vi "DENSITY_txt.vi"(1 "uL/stroke":dbl=5.896, 5 "GUID":string, 7 "derate":dbl=1.0, 9 "Prime":bool=TRUE) -> (3 "density (g/mL)":dbl, 4 "mean":dbl format="%0.4f", 6 "mean 2":dbl format="%0.4f", 8 "standard deviation":dbl format="%0.4f", 10 "standard deviation 2":dbl format="%0.4f", 14 "xxx":bool[](array[boolean]), 15 "Err?":string)   [LabVIEW 2019]
uses:
  <vilib>/Analysis/NI_AALBase.lvlib
panel:
  out "sample (g)":dbl[](array[numeric])
  out "variance 2":dbl format="%0.4f"
  out "InvalidCommandErr? 2":bool
  out "tare (g)":dbl[](array[numeric])
  out "variance":dbl format="%0.4f"
  out "InvalidCommandErr?":bool
  out "log_string":string
  out "SampleVolume (mL)":dbl
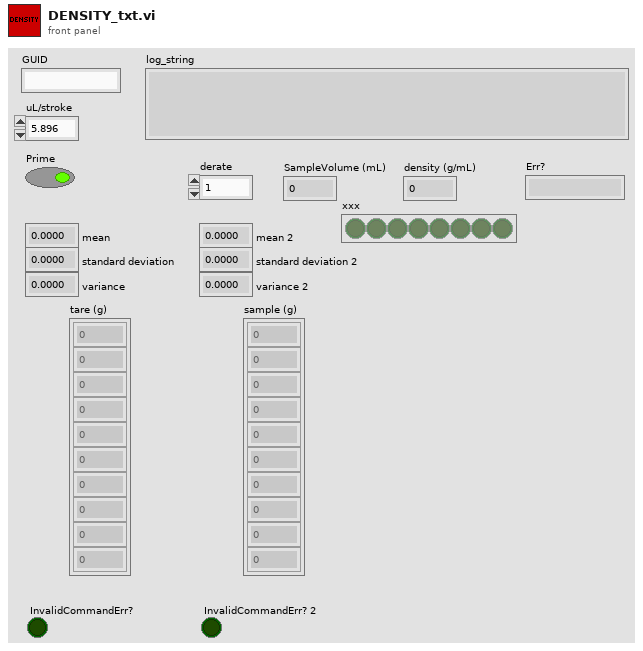
[diagram p1: front panel]
types:
  T1 = enum16{"open", "replace", "create", "open or create", "replace or create", "replace or create with confirmation"}
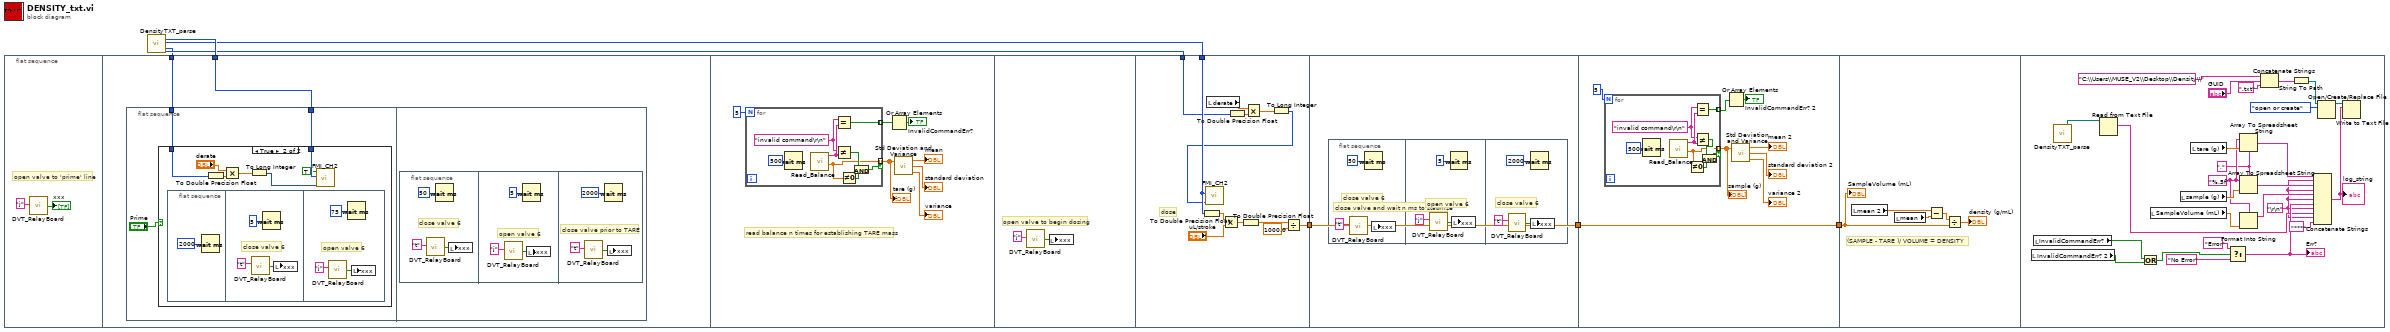
[diagram p0: block diagram]
diagram:
  n1 = flat-sequence {
    tunnel: w4 -> [w11]
    tunnel: w1 -> [w10]
    tunnel: [w66] -> w6
    tunnel: w3 -> [w61]
    tunnel: w2 -> [w58]
    tunnel: [w67] -> w5
    tunnel: w6 -> [w67]
    tunnel: [w84] -> w7
    tunnel: w5 -> [w84]
    tunnel: w7 -> [w94]
    frame #0 {
      # "open valve to 'prime' line"
      n2 = call "DVT_RelayBoard.vi"("write buffer"="j") -> ("Boolean array"=→"xxx":bool[])  [unwired: 3 in, 2 out]
    }
    frame #1 {
      n3 = flat-sequence {
        tunnel: w11 -> [w14]
        tunnel: w10 -> [w12]
        frame #0 {
          n4 = case shown="True" "Prime" {
            tunnel: w14 -> [_ w21]
            tunnel: w12 -> [_ w16]
            frame False {
            }
            frame True {
              n5 = flat-sequence {
                frame #0 {
                  n6 = Wait (ms)(milliseconds to wait=u32 2000) -> ()  [unwired: 1 out]
                }
                frame #1 {
                  # "close valve 6"
                  n7 = call "DVT_RelayBoard.vi"("write buffer"="t") -> ("Boolean array"=w24:bool[])  [unwired: 3 in, 2 out]
                  n8 = Wait (ms)(milliseconds to wait=u32 5) -> ()  [unwired: 1 out]
                  n9 = local write "xxx"(w24) -> ()
                }
                frame #2 {
                  # "open valve 6"
                  n10 = call "DVT_RelayBoard.vi"("write buffer"="j") -> ("Boolean array"=w27:bool[])  [unwired: 3 in, 2 out]
                  n11 = Wait (ms)(milliseconds to wait=u32 75) -> ()  [unwired: 1 out]
                  n12 = local write "xxx"(w27) -> ()
                }
              }
              n13 = To Double Precision Float(number=w16) -> (double precision float=w19:dbl)
              n14 = Multiply(x="derate", y=w19) -> (x*y=w18:dbl)
              n15 = To Long Integer(number=w18) -> (32bit integer=w15:i32)
              n16 = call "FMI_CH2.vi"("RPM"=w15, "Strokes"=w21, "Home Pump"=TRUE) -> ()  [unwired: 4 in, 1 out]
            }
          }
        }
        frame #1 {
          n17 = flat-sequence {
            frame #0 {
              # "close valve 6"
              n18 = call "DVT_RelayBoard.vi"("write buffer"="t") -> ("Boolean array"=w29:bool[])  [unwired: 3 in, 2 out]
              n19 = Wait (ms)(milliseconds to wait=u32 50) -> ()  [unwired: 1 out]
              n20 = local write "xxx"(w29) -> ()
            }
            frame #1 {
              # "open valve 6"
              n21 = call "DVT_RelayBoard.vi"("write buffer"="j") -> ("Boolean array"=w33:bool[])  [unwired: 3 in, 2 out]
              n22 = Wait (ms)(milliseconds to wait=u32 5) -> ()  [unwired: 1 out]
              n23 = local write "xxx"(w33) -> ()
            }
            frame #2 {
              # "close valve prior to TARE"
              n24 = call "DVT_RelayBoard.vi"("write buffer"="t") -> ("Boolean array"=w35:bool[])  [unwired: 3 in, 2 out]
              n25 = Wait (ms)(milliseconds to wait=u32 2000) -> ()  [unwired: 1 out]
              n26 = local write "xxx"(w35) -> ()
            }
          }
        }
      }
    }
    frame #2 {
      # "read balance n times for establishing TARE mass"
      n27 = for {
        N: 5 -> [_]
        tunnel: [w45] -> w44 mode=indexing if=w46
        tunnel: [w49] -> w42 mode=indexing
        w50 = "invalid command\r\n"
        n28 = Wait (ms)(milliseconds to wait=u32 500) -> ()  [unwired: 1 out]
        n29 = call "Read_Balance.vi"() -> ("string"=w51:string, "Mass (dbl)"=w45:dbl)  [unwired: 3 in, 3 out]
        n30 = Equal?(x=w50, y=w51) -> (x = y?=w49:bool)
        n31 = Not Equal?(x=w50, y=w51) -> (x != y?=w47:bool)
        n32 = Not Equal To 0?(x=w45) -> (x != 0?=w48:bool)
        n33 = And(x=w47, y=w48) -> (x .and. y?=w46:bool)
      }
      "tare (g)" <- w44
      n34 = Or Array Elements(Boolean array=w42) -> (logical OR=→"InvalidCommandErr?":bool)
      n35 = call <vilib>:"Std Deviation and Variance.vi"("X"=w44) -> ("mean"=→"mean":dbl, "standard deviation"=→"standard deviation":dbl, "variance"=→"variance":dbl)  [unwired: 1 in]
    }
    frame #3 {
      # "open valve to begin dosing"
      n36 = call "DVT_RelayBoard.vi"("write buffer"="j") -> ("Boolean array"=w53:bool[])  [unwired: 3 in, 2 out]
      n37 = local write "xxx"(w53) -> ()
    }
    frame #4 {
      # "dose"
      n38 = To Double Precision Float(number=w61) -> (double precision float=w60:dbl)
      n39 = local read "derate"() -> (w55:dbl)
      n40 = Multiply(x=w60, y="uL/stroke") -> (x*y=w62:dbl)
      n41 = To Double Precision Float(number=w58) -> (double precision float=w59:dbl)
      n42 = To Double Precision Float(number=w62) -> (double precision float=w63:dbl)
      n43 = Multiply(x=w55, y=w59) -> (x*y=w57:dbl)
      n44 = To Long Integer(number=w57) -> (32bit integer=w56:i32)
      n45 = call "FMI_CH2.vi"("RPM"=w56, "Strokes"=w61) -> ()  [unwired: 5 in, 1 out]
      n46 = Divide(x=w63, y=1000.0) -> (x/y=w66:dbl)
    }
    frame #5 {
      # "close valve and wait n ms to stabilize"
      n47 = flat-sequence {
        frame #0 {
          # "close valve 6"
          n48 = call "DVT_RelayBoard.vi"("write buffer"="t") -> ("Boolean array"=w69:bool[])  [unwired: 3 in, 2 out]
          n49 = Wait (ms)(milliseconds to wait=u32 50) -> ()  [unwired: 1 out]
          n50 = local write "xxx"(w69) -> ()
        }
        frame #1 {
          # "open valve 6"
          n51 = call "DVT_RelayBoard.vi"("write buffer"="j") -> ("Boolean array"=w72:bool[])  [unwired: 3 in, 2 out]
          n52 = Wait (ms)(milliseconds to wait=u32 5) -> ()  [unwired: 1 out]
          n53 = local write "xxx"(w72) -> ()
        }
        frame #2 {
          # "close valve 6"
          n54 = call "DVT_RelayBoard.vi"("write buffer"="t") -> ("Boolean array"=w74:bool[])  [unwired: 3 in, 2 out]
          n55 = Wait (ms)(milliseconds to wait=u32 2000) -> ()  [unwired: 1 out]
          n56 = local write "xxx"(w74) -> ()
        }
      }
    }
    frame #6 {
      n57 = for {
        N: 5 -> [_]
        tunnel: [w85] -> w83 mode=indexing if=w87
        tunnel: [w89] -> w81 mode=indexing
        w90 = "invalid command\r\n"
        n58 = Wait (ms)(milliseconds to wait=u32 500) -> ()  [unwired: 1 out]
        n59 = call "Read_Balance.vi"() -> ("string"=w91:string, "Mass (dbl)"=w85:dbl)  [unwired: 3 in, 3 out]
        n60 = Not Equal To 0?(x=w85) -> (x != 0?=w86:bool)
        n61 = Equal?(x=w90, y=w91) -> (x = y?=w89:bool)
        n62 = Not Equal?(x=w90, y=w91) -> (x != y?=w88:bool)
        n63 = And(x=w88, y=w86) -> (x .and. y?=w87:bool)
      }
      "sample (g)" <- w83
      n64 = Or Array Elements(Boolean array=w81) -> (logical OR=→"InvalidCommandErr? 2":bool)
      n65 = call <vilib>:"Std Deviation and Variance.vi"("X"=w83) -> ("mean"=→"mean 2":dbl, "standard deviation"=→"standard deviation 2":dbl, "variance"=→"variance 2":dbl)  [unwired: 1 in]
    }
    frame #7 {
      # "(SAMPLE - TARE )/ VOLUME = DENSITY"
      n66 = local read "mean 2"() -> (w97:dbl)
      n67 = local read "mean"() -> (w96:dbl)
      n68 = Subtract(x=w97, y=w96) -> (x-y=w95:dbl)
      n69 = Divide(x=w95, y=w94) -> (x/y=→"density (g/mL)":dbl)
      "SampleVolume (mL)" <- w94
    }
    frame #8 {
      w98 = "\r\n"
      w108 = "," ("delimiter (Tab)")
      w109 = "%.5f" ("format (%.3f)")
      n70 = local read "InvalidCommandErr? 2"() -> (w102:bool)
      n71 = local read "InvalidCommandErr?"() -> (w101:bool)
      n72 = call "DensityTXT_parse.vi"() -> ("file path (dialog if empty)"=w100:path)  [unwired: 13 in, 6 out]
      n73 = Read from Text File(file (use dialog)=w100) -> (text=w99:string)  [unwired: 3 in, 3 out]
      n74 = Or(x=w101, y=w102) -> (x .or. y?=w103:bool)
      n75 = local read "SampleVolume (mL)"() -> (w113:dbl)
      n76 = local read "sample (g)"() -> (w114:dbl[])
      n77 = local read "tare (g)"() -> (w116:dbl[])
      n78 = Select(t="Error" ("string"), s=w103, f="No Error") -> (s? t:f=w106:string)
      "Err?" <- w106
      n79 = Array To Spreadsheet String(delimiter (Tab)=w108, array=w116, 3:w109) -> (spreadsheet string=w115:string)
      n80 = Array To Spreadsheet String(delimiter (Tab)=w108, array=w114, 3:w109) -> (spreadsheet string=w112:string)
      n81 = Format Into String(format string=w109, w113) -> (resulting string=w111:string)  [unwired: 2 in, 1 out]
      n82 = Concatenate Strings("C:\\Users\\MUSE_V2\\Desktop\\Density\\", "GUID", ".txt" ("string")) -> (w121:string)
      n83 = String To Path(string=w121) -> (path=w119:path)
      n84 = Concatenate Strings(w115, w98, w112, w98, w111, w98, w106, w98, w99, w98, "***" ("string")) -> (w110:string)
      "log_string" <- w110
      n85 = Open/Create/Replace File(file path (use dialog)=w119, operation (0:open)=T1."open or create") -> (refnum out=w120:refnum<file>)  [unwired: 4 in, 2 out]
      n86 = Write to Text File(file (use dialog)=w120, text=w110) -> ()  [unwired: 2 in, 3 out]
    }
  }
  n87 = call "DensityTXT_parse.vi"() -> ("Strokes_Pr2"=w4:i32, "Strokes_Dose"=w3:i32, "RPM_Pr2"=w1:i32, "RPM_Dose"=w2:i32)  [unwired: 13 in, 3 out]
